vi "Get True-False String.vi"(1 "Input":bool) -> (0 "True/False String":string)   [LabVIEW 2020, in "Output Sequencer.lvlib" / "Settings UI.lvclass"]
uses:
  Settings UI.lvclass
  Output Sequencer/Globals/Global Strings.vi
  Output Sequencer/Output Sequencer.lvclass
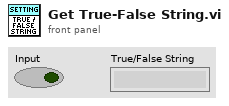
[diagram p1: front panel]
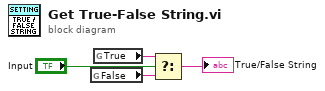
[diagram p0: block diagram]
diagram:
  n1 = global read "Global Strings.vi" "False"() -> (w4:string)
  n2 = global read "Global Strings.vi" "True"() -> (w3:string)
  n3 = Select(t=w3, s="Input", f=w4) -> (s? t:f=→"True/False String":string)
